vi "Azimuth.vi"() -> ()   [LabVIEW 2013]
doc: "This example performs a serial port write and a serial port read. The parameters set for the serial port must match the parameters of the connected instrument or device. The VISA Configure Serial Port VI sets the configuration parameters. The front panel displays the controls used to configure the basic parameters, such as baud rate, data bits, and parity. The VI passes the VISA resource name to other VIs that perform operations on that VISA resource. The VISA Write function sends a command to the serial device and the VISA Read function returns data based on the command. The VISA Close function then closes the reference to the serial device. It is important to close the reference; otherwise, further communication through that port might not be possible."
uses:
  C:/Program Files (x86)/National Instruments/LabVIEW 2013/examples/Instrument IO/Serial/support/Serial - Settings.ctl
  <vilib>/Instr/_visa.llb/VISA Configure Serial Port (Instr).vi
panel:
  out "Map 2":cluster{dbl[], dbl[]}[](graph)
  out "% of garbage":dbl
  out "Not garbage packets":u32=19
  out "Garbage packets":u32=19
  in  "Bytes to read":u32=19
  out "Map":cluster{dbl[], dbl[]}[](graph)
  out "Encoder2":u16
  out "Encoder1":u16
  out "IR1":u16
  out "IR2":u16
  out "String to U16":u16[](array[numeric])
  in  "?":bool
  in  "Serial Settings":T1={"baud rate"=9600, "data bits"=8, "parity"=enum."None", "stop bits"=10, "flow control"=0} {"flow control" items=["None"=0, "XON/XOFF"=1, "RTS/CTS"=2, "DTR/DSR"=4]; "stop bits" items=["1.0"=10, "1.5"=15, "2.0"=20]; "data bits" min=5 max=8 step=1; "baud rate" items=["75"=75, "110"=110, "134"=134, "150"=150, "300"=300, "600"=600, "1200"=1200, "1800"=1800, "2400"=2400, "4800"=4800, "7200"=7200, "9600"=9600, "14400"=14400, "19200"=19200, "28800"=28800, "38400"=38400, "56000"=56000, "57600"=57600, "115200"=115200, "128000"=128000, "230400"=230400]}
  out "Bytes read":u32
  in  "delay before read (ms)":u32=25
  out "Response":string
  in  "VISA resource name":refnum<visa-resource-name>="COM1"
  # "Azimuth"
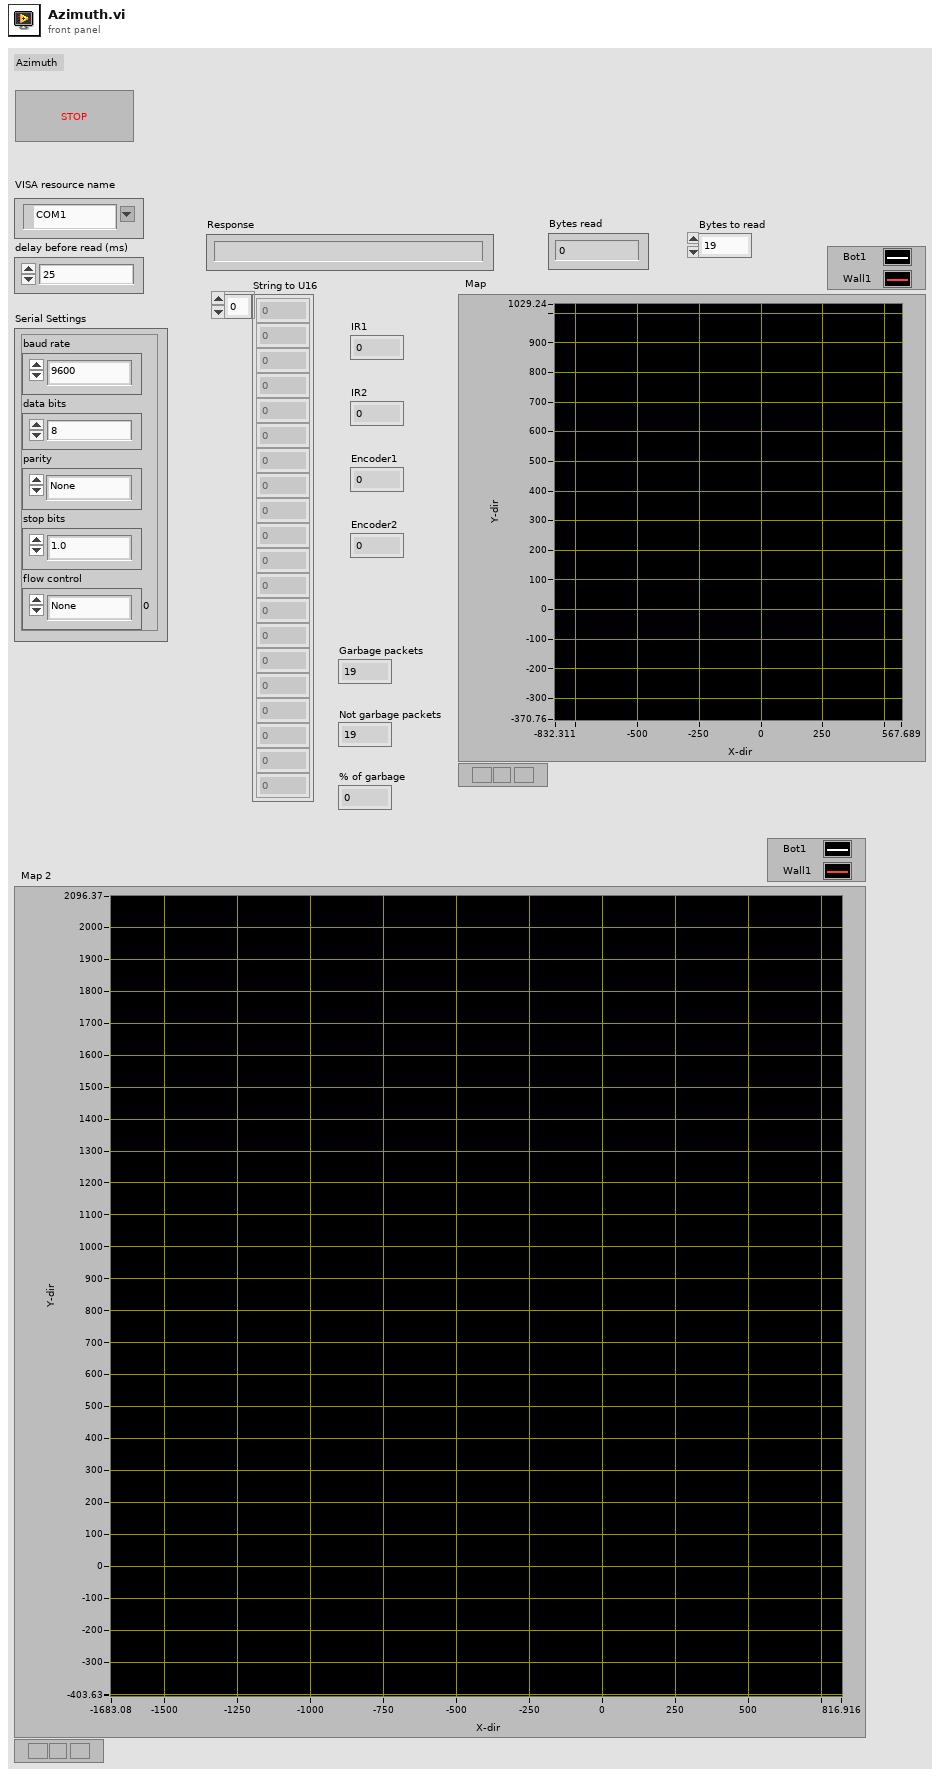
[diagram p1: front panel]
types:
  T1 = typedef "Serial - Settings.ctl" = cluster{"baud rate":u32, "data bits":u16, "parity":enum16{"None", "Odd", "Even", "Mark", "Space"}, "stop bits":u16, "flow control":u16}
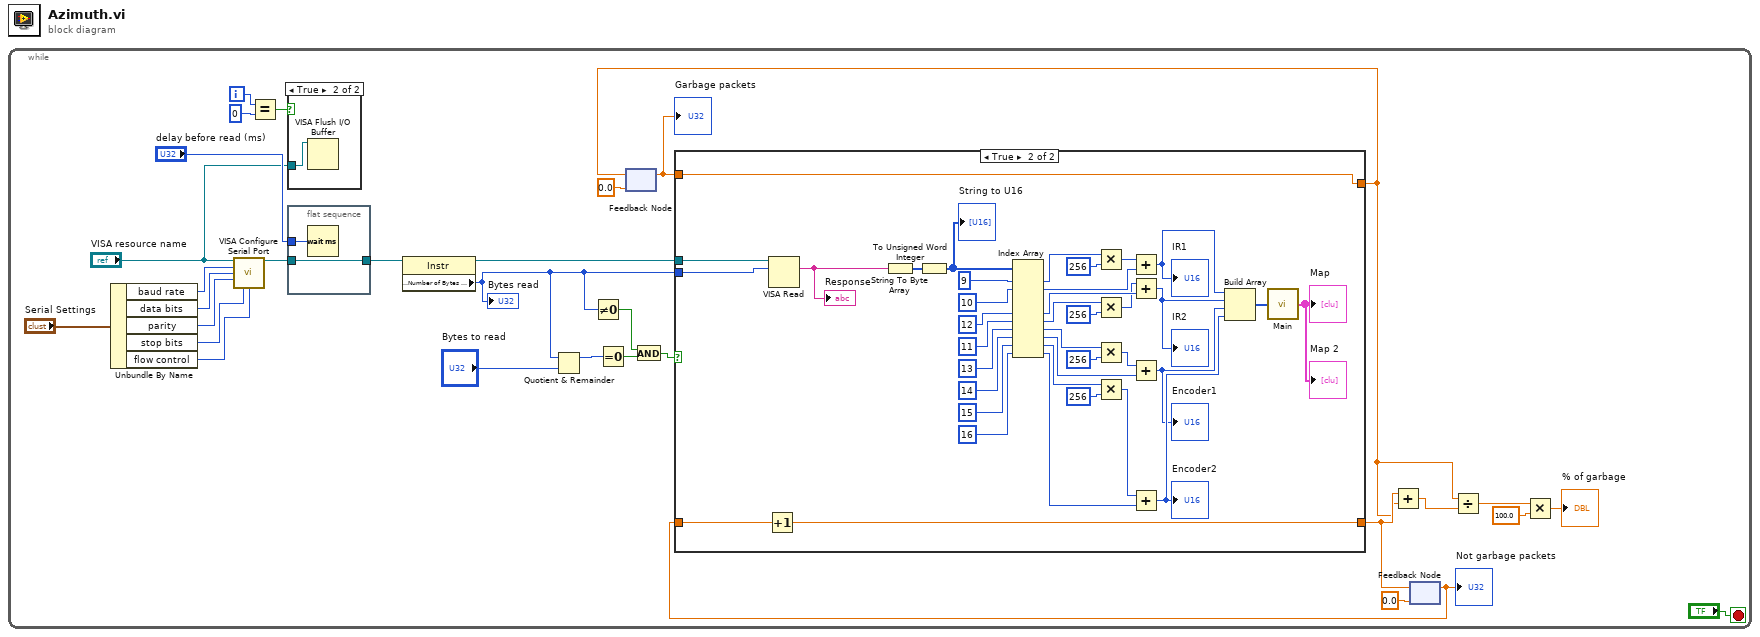
[diagram p0: block diagram]
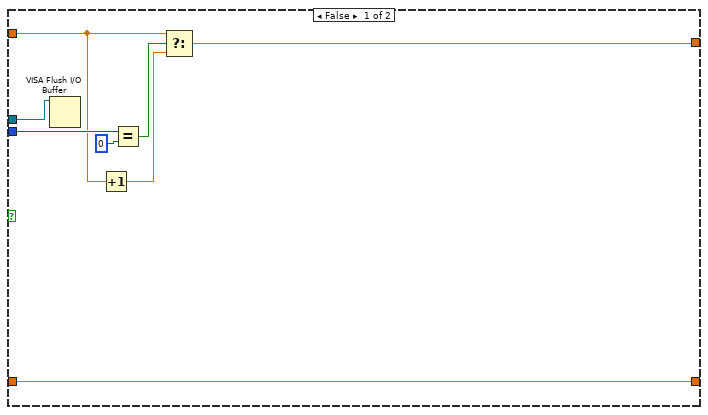
[diagram p2: hidden frame]
diagram:
  n1 = while {
    i -> [w21]
    stop <- "?" stop-if-true
    n2 = Unbundle By Name("Serial Settings") -> ("baud rate"=w29:u32, "data bits"=w28:u16, "parity"=w27:enum16{"None", "Odd", "Even", "Mark", "Space"}, "stop bits"=w26:u16, "flow control"=w25:u16)
    n3 = call-poly "VISA Configure Serial Port"("VISA resource name"="VISA resource name", "baud rate (9600)"=w29, "data bits (8)"=w28, "parity (0:none)"=w27, "stop bits (10: 1 bit)"=w26, "flow control (0:none)"=w25) -> ("VISA resource name out"=w24:refnum<visa-resource-name>)  [unwired: 3 in, 6 out]
    n4 = Equal?(x=w21, y=0) -> (x = y?=w19:bool)
    n5 = case shown="True" w19 {
      tunnel: "VISA resource name" -> [_ w78]
      frame False {
      }
      frame True {
        n6 = VISA Flush I/O Buffer(VISA resource name=w78) -> ()  [unwired: 2 in, 2 out]
      }
    }
    n7 = flat-sequence {
      tunnel: w24 -> [w79]
      tunnel: [w79] -> w23
      tunnel: "delay before read (ms)" -> [w80]
      frame #0 {
        n8 = Wait (ms)(milliseconds to wait=w80) -> ()  [unwired: 1 out]
      }
    }
    n9 = property class="Instr"(reference=w23) -> (reference out=w17:refnum<visa-resource-name>, "Serial Settings:Number of Bytes at Serial Port"=w6:u32)  [unwired: 1 in, 1 out]
    "Bytes read" <- w6
    n10 = Quotient & Remainder(x=w6, y="Bytes to read") -> (x-y*floor(x/y)=w8:u32)  [unwired: 1 out]
    n11 = Not Equal To 0?(x=w6) -> (x != 0?=w5:bool)
    n12 = Equal To 0?(x=w8) -> (x = 0?=w7:bool)
    n13 = feedback #1(0.0) -> (w16:dbl)
    "Garbage packets" <- w16
    n14 = And(x=w5, y=w7) -> (x .and. y?=w4:bool)
    n15 = feedback #2(0.0) -> (w14:dbl)
    "Not garbage packets" <- w14
    n16 = case shown="True" w4 {
      tunnel: w6 -> [w34 w45]
      tunnel: w17 -> [w39 w44]
      tunnel: [w32 w43] -> w2
      tunnel: w16 -> [w33 w43]
      tunnel: w14 -> [w38 w42]
      tunnel: [w38 w41] -> w3
      frame False {
        n17 = VISA Flush I/O Buffer(VISA resource name=w39) -> ()  [unwired: 2 in, 2 out]
        n18 = Increment(x=w33) -> (x+1=w37:dbl)
        n19 = Equal?(x=w34, y=u32 0) -> (x = y?=w35:bool)
        n20 = Select(t=w33, s=w35, f=w37) -> (s? t:f=w32:dbl)
      }
      frame True {
        n21 = Increment(x=w42) -> (x+1=w41:dbl)
        n22 = VISA Read(VISA resource name=w44, byte count=w45) -> (read buffer=w47:string)  [unwired: 1 in, 3 out]
        "Response" <- w47
        n23 = String To Byte Array(string=w47) -> (unsigned byte array=w48:u8[])
        n24 = To Unsigned Word Integer(number=w48) -> (unsigned 16bit integer=w46:u16[])
        "String to U16" <- w46
        n25 = Index Array(array=w46, index #1=9 ("index"), index #2=10 ("index"), index #5=12, index #6=11 ("index"), index #7=13 ("index"), index #8=14 ("index"), index #9=15 ("index"), index #10=16 ("index")) -> (element #1=w56:u16, element #2=w59:u16, element #5=w53:u16, element #6=w51:u16, element #7=w64:u16, element #8=w65:u16, element #9=w71:u16, element #10=w72:u16)  [unwired: 2 in, 2 out]
        n26 = Multiply(x=w56, y=u16 256) -> (x*y=w58:u16)
        n27 = Multiply(x=w51, y=u16 256) -> (x*y=w49:u16)
        n28 = Multiply(x=w64, y=u16 256) -> (x*y=w60:u16)
        n29 = Multiply(x=w71, y=u16 256) -> (x*y=w70:u16)
        n30 = Add(x=w58, y=w59) -> (x+y=w73:u16)
        "IR1" <- w73
        n31 = Add(x=w49, y=w53) -> (x+y=w74:u16)
        "IR2" <- w74
        n32 = Add(x=w60, y=w65) -> (x+y=w75:u16)
        "Encoder1" <- w75
        n33 = Add(x=w70, y=w72) -> (x+y=w76:u16)
        "Encoder2" <- w76
        n34 = Build Array(w73, w74, w75, w76) -> (w77:u16[])
        n35 = call "Main.vi"("bot array"=w77) -> ("XY array"=→"Map" →"Map 2":cluster{dbl[], dbl[]}[])
      }
    }
    n36 = feedback-in #1(w2) -> ()
    n37 = Add(x=w3, y=w2) -> (x+y=w1:dbl)
    n38 = feedback-in #2(w3) -> ()
    n39 = Divide(x=w2, y=w1) -> (x/y=w12:dbl)
    n40 = Multiply(x=w12, y=100.0) -> (x*y=→"% of garbage":dbl)
  }
